vi "JanPID_auton.vi"(8 "Scaling":dbl=1.0, 9 "Feedback":dbl, 10 "Setpoint":dbl, 11 "P":dbl=0.05) -> (2 "Error":dbl, 3 "Motor Output":dbl)   [LabVIEW 2011]
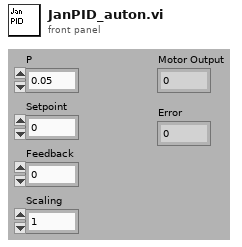
[diagram p1: front panel]
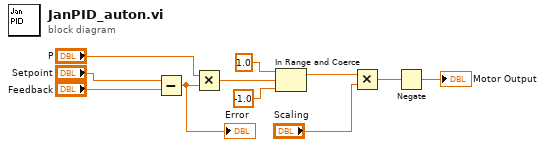
[diagram p0: block diagram]
diagram:
  n1 = Subtract(x="Setpoint", y="Feedback") -> (x-y=w1:dbl)
  "Error" <- w1
  n2 = Multiply(x="P", y=w1) -> (x*y=w8:dbl)
  n3 = In Range and Coerce(upper limit=1.0, x=w8, lower limit=-1.0) -> (coerced(x)=w3:dbl)  [unwired: 1 out]
  n4 = Multiply(x=w3, y="Scaling") -> (x*y=w4:dbl)
  n5 = Negate(x=w4) -> (-x=→"Motor Output":dbl)
